vi "PRIME Detector Close.vi"(8 "error in (no error)":errorcluster, 11 "connection ID":refnum<k5>[](array[refnum])) -> (0 "error out":errorcluster, 3 "connection ID out":refnum<k5>[](array[refnum]))   [LabVIEW 2024, in "PRIME Detector.lvclass"]
uses:
  PRIME Detector.lvclass
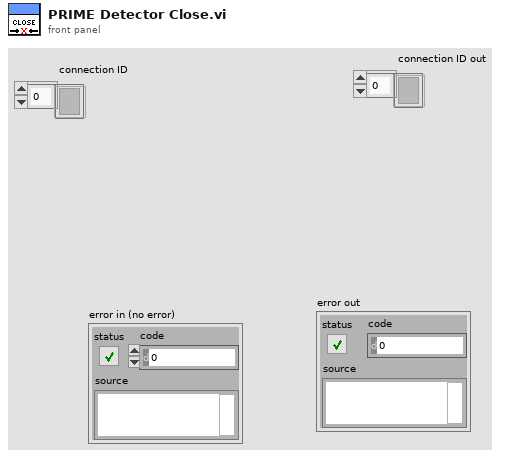
[diagram p1: front panel]
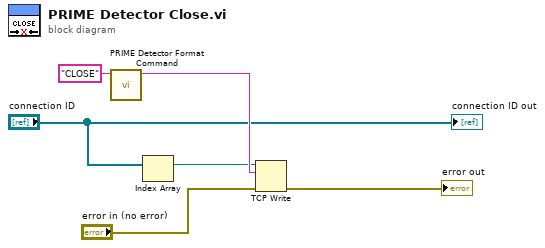
[diagram p0: block diagram]
diagram:
  n1 = call "PRIME Detector Format Command.vi"("Command"="CLOSE") -> ("TCP String"=w5:string)  [unwired: 10 in]
  n2 = Index Array(array="connection ID") -> (element=w2:refnum<k5>)  [unwired: 1 in]
  n3 = TCP Write(connection ID=w2, data in=w5, error in (no error)="error in (no error)") -> (error out=→"error out":errorcluster)  [unwired: 1 in, 2 out]
  "connection ID out" <- "connection ID"
